vi "coefficients.vi"(10 "k-constant":dbl=3.2, 11 "Numeric":i32=32) -> (2 "cosine":i16[](array[numeric])=[71, 0, -71, -100, -71, 0, 71, 100, 71, 0, -71, -100, -71, 0, 71, 100, 71, 0, -71, -100, -71, 0, 71, 100, 71, 0, -71, -100, -71, 0, 71, 100], 3 "sine":i16[](array[numeric])=[71, 100, 71, 0, -71, -100, -71, 0, 71, 100, 71, 0, -71, -100, -71, 0, 71, 100, 71, 0, -71, -100, -71, 0, 71, 100, 71, 0, -71, -100, -71, 0])   [LabVIEW 2017]
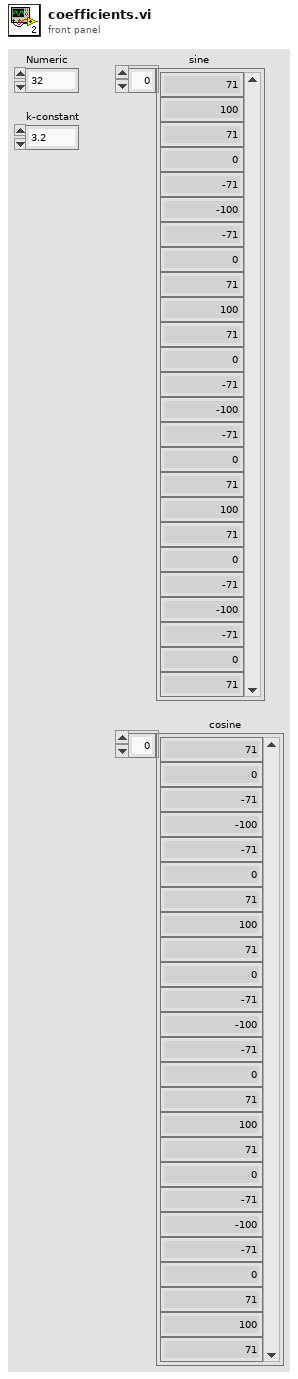
[diagram p1: front panel]
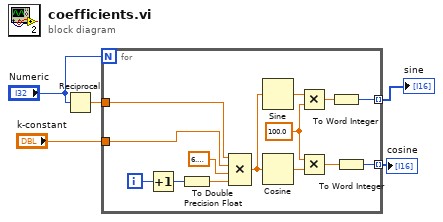
[diagram p0: block diagram]
diagram:
  n1 = Reciprocal(x="Numeric") -> (1/x=w2:dbl)
  n2 = for {
    N: "Numeric" -> [_]
    tunnel: w2 -> [w16]
    tunnel: [w9] -> w4 mode=indexing
    tunnel: [w8] -> w3 mode=indexing
    tunnel: "k-constant" -> [w6]
    i -> [w18]
    w13 = 100.0 ("y")
    n3 = Increment(x=w18) -> (x+1=w15:i32)
    n4 = To Double Precision Float(number=w15) -> (double precision float=w17:dbl)
    n5 = Compound Arithmetic op=MULTIPLY(w16, w6, 6.283185307179586, w17) -> (w7:dbl)
    n6 = Sine(x=w7) -> (sin(x)=w14:dbl)
    n7 = Cosine(x=w7) -> (cos(x)=w12:dbl)
    n8 = Multiply(x=w14, y=w13) -> (x*y=w11:dbl)
    n9 = Multiply(x=w13, y=w12) -> (x*y=w10:dbl)
    n10 = To Word Integer(number=w11) -> (16bit integer=w9:i16)
    n11 = To Word Integer(number=w10) -> (16bit integer=w8:i16)
  }
  "sine" <- w4
  "cosine" <- w3
